vi "ClearHardware.vi"(3 "error in (no error)":errorcluster, 5 "Tasks Out":refnum<k21>[](array[refnum])) -> (0 "error out":errorcluster)   [LabVIEW 2012]
doc: "This vi clears the hardware used to run the Rubidium experiment. (The analog output boards and the counter if we are synching to the camera.)\n\nIt's inputs:\n1) a cluster of the 3 task ID's and the synch to camera boolean\n3) error in\nIt's output\n1) error out."
uses:
  <vilib>/DAQmx/write.llb/DAQmx Write (Analog 1D DBL NChan 1Samp).vi
  <vilib>/DAQmx/miscellaneous.llb/DAQmx Fill In Error Info.vi
  Pulseblaster/PulseBlaster.lvlib
panel:
  in  "Set to zero":bool
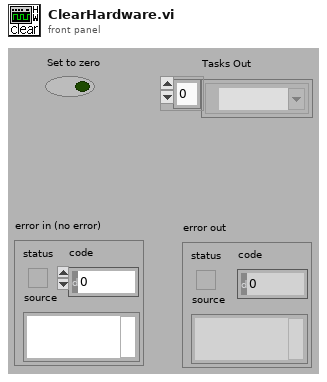
[diagram p1: front panel]
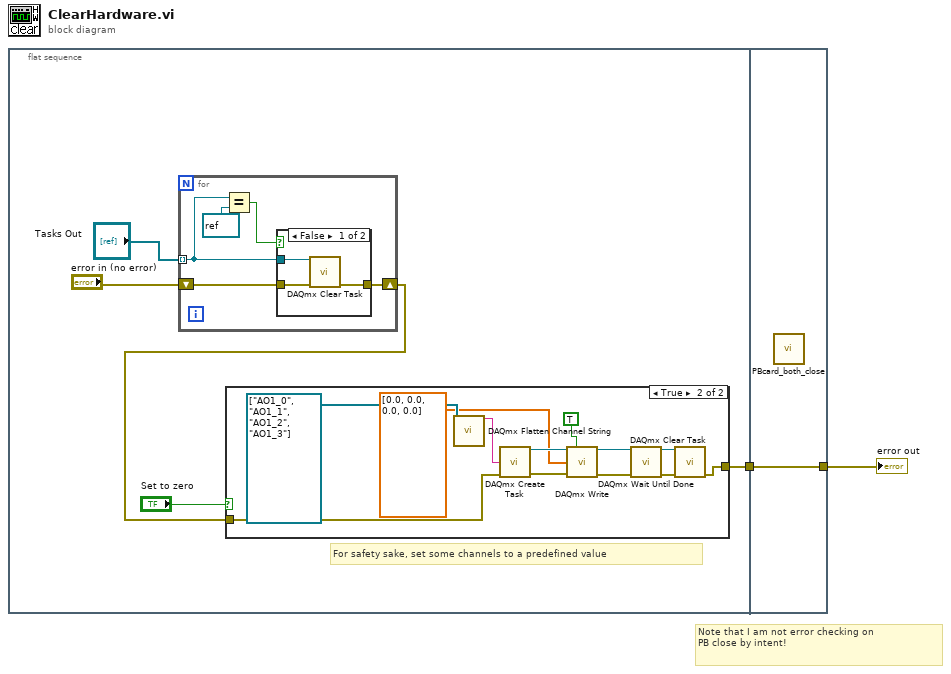
[diagram p0: block diagram]
diagram:
  # "Note that I am not error checking on\nPB close by intent!"
  n1 = flat-sequence {
    tunnel: [w5] -> w1
    tunnel: [w30] -> w2
    tunnel: w1 -> [w30]
    frame #0 {
      # "For safety sake, set some channels to a predefined value"
      n2 = for {
        shift-right: [w9] -> w4
        shift-left: "error in (no error)" -> [w12]
        tunnel: "Tasks Out" -> [w8] mode=indexing
        n3 = Equal?(x=w8, y=refnum<k21> refnum ("Name")) -> (x = y?=w10:bool)
        n4 = case shown="False" w10 {
          tunnel: w12 -> [w15 w16]
          tunnel: [w14 w16] -> w9
          tunnel: w8 -> [w13 _]
          frame False {
            n5 = call <vilib>:"DAQmx Clear Task.vi"("task in"=w13, "error in"=w15) -> ("error out"=w14:errorcluster)  [unwired: 13 out]
          }
          frame True {
          }
        }
      }
      n6 = case shown="True" "Set to zero" {
        tunnel: w4 -> [w17 w21]
        tunnel: [w17 w27] -> w5
        frame False {
        }
        frame True {
          n7 = call <vilib>:"DAQmx Flatten Channel String.vi"("names in"=refnum<k21>[] ["AO1_0", "AO1_1", "AO1_2", "AO1_3"]) -> ("names out"=w20:string)  [unwired: 1 in, 13 out]
          n8 = call <vilib>:"DAQmx Create Task.vi"("global virtual channels"=w20, "error in"=w21) -> ("task out"=w26:refnum<k21>, "error out"=w25:errorcluster)  [unwired: 3 in, 9 out]
          n9 = call-poly <vilib>:"DAQmx Write.vi"("task/channels in"=w26, "auto start"=TRUE, "data"=dbl[] [0.0, 0.0, 0.0, 0.0], "error in"=w25) -> ("task out"=w23:refnum<k21>, "error out"=w22:errorcluster)  [unwired: 10 out]
          n10 = call <vilib>:"DAQmx Wait Until Done.vi"("task/channels in"=w23, "error in"=w22) -> ("task out"=w29:refnum<k21>, "error out"=w28:errorcluster)  [unwired: 1 in, 11 out]
          n11 = call <vilib>:"DAQmx Clear Task.vi"("task in"=w29, "error in"=w28) -> ("error out"=w27:errorcluster)  [unwired: 13 out]
        }
      }
    }
    frame #1 {
      n12 = call "PBcard_both_close.vi"() -> ()  [unwired: 1 in, 2 out]
    }
  }
  "error out" <- w2
